vi "Z900_navX_InternalOpen.vi"(8 "error in":errorcluster, 11 "navX Device":T1={"Interface"={"Protocol"=enum."SERIAL", "Update Rate (4Hz-60Hz)"=4, "navX Open TypeDef"=variant}, "Notify Packet"=refnum, "Loop VI Refnum"=refnum} {"Interface"."Update Rate (4Hz-60Hz)" min=4 max=60 step=1}) -> (0 "error out":errorcluster, 2 "Interface TypeDefs":T3 {"I2CDevRef"."Device Address" format="%.0x"}, 3 "navX Device":T1={"Interface"={"Protocol"=enum."SERIAL", "Update Rate (4Hz-60Hz)"=4, "navX Open TypeDef"=variant}, "Notify Packet"=refnum, "Loop VI Refnum"=refnum} {"Interface"."Update Rate (4Hz-60Hz)" min=4 max=60 step=1})   [LabVIEW 2014, in "navX Library v2.lvlib"]
uses:
  navX Library v2.lvlib
  TypeDefs/Z900_navX_DeviceTypeDef.ctl
  TypeDefs/Z900_navX_ProtocolTypeDef.ctl
  TypeDefs/Z900_navX_NotifyPacketTypeDef.ctl
  TypeDefs/Z900_navX_ActionTypeDef.ctl
  TypeDefs/Z900_navX_InterfaceTypeDef.ctl
  <vilib>/Rock Robotics/WPI/SerialPort/WPI_SerialPortRef.ctl
  <vilib>/Rock Robotics/WPI/I2C/WPI_I2CDevRef.ctl
  <vilib>/Rock Robotics/SystemInterfaces/Typedef/FPGA_TypedefDigitalModule.ctl
  <vilib>/Rock Robotics/SystemInterfaces/i2clib/i2c_bus.ctl
  <vilib>/Rock Robotics/WPI/SPI/WPI_SPIDevRef.ctl
  <vilib>/Rock Robotics/SystemInterfaces/spilib/spi_bus.ctl
  TypeDefs/navX Open TypeDefs/Z900_navX_SerialOpenTypeDef.ctl
  NI WPI/WPI_SerialPort_USB.ctl
  TypeDefs/navX Open TypeDefs/Z900_navX_I2COpenTypeDef.ctl
  TypeDefs/navX Open TypeDefs/Z900_navX_SPIOpenTypeDef.ctl
  NI WPI/NI WPI Serial USB.lvlib
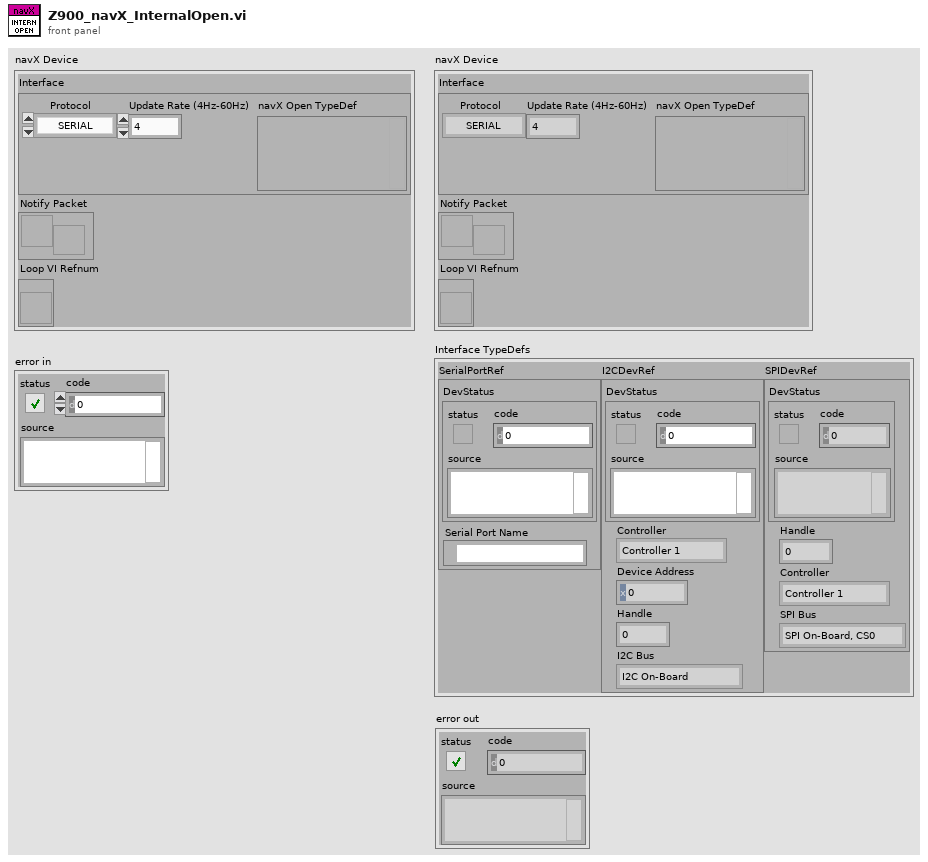
[diagram p1: front panel]
types:
  T1 = typedef "navX Library v2.lvlib/Z900_navX_DeviceTypeDef.ctl" = cluster{"Interface":cluster{"Protocol":T2, "Update Rate (4Hz-60Hz)":u8, "navX Open TypeDef":variant}, "Notify Packet":refnum<notifier>, "Loop VI Refnum":refnum<vi>}
  T2 = typedef "navX Library v2.lvlib/Z900_navX_ProtocolTypeDef.ctl" = enum16{"SERIAL", "I2C", "SPI"}
  T3 = typedef "navX Library v2.lvlib/Z900_navX_InterfaceTypeDef.ctl" = cluster{"SerialPortRef":T4, "I2CDevRef":T5, "SPIDevRef":T8}
  T4 = typedef "WPI_SerialPortRef.ctl" = cluster{"DevStatus":errorcluster, "Serial Port Name":refnum<visa-resource-name>}
  T5 = typedef "WPI_I2CDevRef.ctl" = cluster{"DevStatus":errorcluster, "Controller":T6, "Device Address":u8, "Handle":i32, "I2C Bus":T7}
  T6 = typedef "FPGA_TypedefDigitalModule.ctl" = enum16{"Controller 1"}
  T7 = typedef "i2c_bus.ctl" = enum16{"I2C On-Board", "I2C MXP", "Invalid"}
  T8 = typedef "WPI_SPIDevRef.ctl" = cluster{"DevStatus":errorcluster, "Handle":i32, "Controller":T6, "SPI Bus":T9}
  T9 = typedef "spi_bus.ctl" = enum16{"SPI On-Board, CS0", "SPI On-Board, CS1", "SPI On-Board, CS2", "SPI On-Board, CS3", "SPI MXP", "Invalid"}
  T10 = typedef "navX Library v2.lvlib/Z900_navX_SerialOpenTypeDef.ctl" = cluster{"Serial Port":T11, "Raw Data":bool}
  T11 = typedef "NI WPI Serial USB.lvlib/WPI_SerialPort_USB.ctl" = enum16{"Onboard RS-232", "MXP TTL", "USB"}
  T12 = typedef "navX Library v2.lvlib/Z900_navX_I2COpenTypeDef.ctl" = cluster{"I2C Bus":T7}
  T13 = typedef "navX Library v2.lvlib/Z900_navX_SPIOpenTypeDef.ctl" = cluster{"SPI Bus":T9}
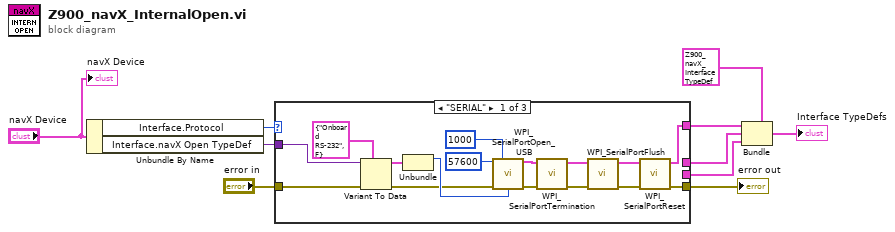
[diagram p0: block diagram]
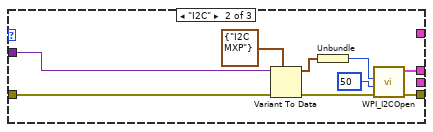
[diagram p2: hidden frame]
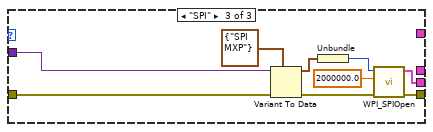
[diagram p3: hidden frame]
diagram:
  n1 = Unbundle By Name("navX Device") -> ("Interface.Protocol"=w7:T2, "Interface.navX Open TypeDef"=w6:variant)
  n2 = case shown="\"SERIAL\"" w7 {
    tunnel: w6 -> [w26 w34 w43]
    tunnel: [w14 _ _] -> w10
    tunnel: [w13 w30 w39] -> w5
    tunnel: [_ w29 _] -> w9
    tunnel: [_ _ w38] -> w8
    tunnel: "error in" -> [w12 w27 w37]
    frame "SERIAL" {
      n3 = Variant To Data(error in=w12, type=T10 {"Serial Port"=enum."Onboard RS-232", "Raw Data"=FALSE} ("navX Serial Open"), Variant=w26) -> (data=w24:T10, error out=w11:errorcluster)
      n4 = Unbundle(w24) -> ("Serial Port"=w23:T11)  [unwired: 1 out]
      n5 = call "WPI_SerialPortOpen_USB.vi"("Baud Rate"=u32 57600, "Timeout Value (ms)"=u32 1000, "error in (no error)"=w11, "Serial Port"=w23) -> ("SerialPortRef"=w16:T4, "error out"=w15:errorcluster)  [unwired: 10 in]
      n6 = call <vilib>:"WPI_SerialPortTermination.vi"("error in (no error)"=w15, "SerialPortRef"=w16) -> ("error out"=w20:errorcluster, "SerialPortRef"=w19:T4)  [unwired: 8 in]
      n7 = call <vilib>:"WPI_SerialPortFlush.vi"("error in (no error)"=w20, "SerialPortRef"=w19) -> ("error out"=w17:errorcluster, "SerialPortRef"=w18:T4)  [unwired: 8 in]
      n8 = call <vilib>:"WPI_SerialPortReset.vi"("error in (no error)"=w17, "SerialPortRef"=w18) -> ("error out"=w13:errorcluster, "SerialPortRef"=w14:T4)  [unwired: 8 in]
    }
    frame "I2C" {
      n9 = Variant To Data(error in=w27, type=T12 {"I2C Bus"=enum."I2C MXP"} ("navX I2C Open"), Variant=w34) -> (data=w35:T12, error out=w28:errorcluster)
      n10 = Unbundle(w35) -> ("I2C Bus"=w32:T7)
      n11 = call <vilib>:"WPI_I2COpen.vi"("error in"=w28, "Device Address"=u8 50, "I2C Bus"=w32) -> ("error out"=w30:errorcluster, "I2CDevRef"=w29:T5)  [unwired: 7 in]
    }
    frame "SPI" {
      n12 = Variant To Data(error in=w37, type=T13 {"SPI Bus"=enum."SPI MXP"} ("navX SPI Open"), Variant=w43) -> (data=w44:T13, error out=w36:errorcluster)
      n13 = Unbundle(w44) -> ("SPI Bus"=w41:T9)
      n14 = call <vilib>:"WPI_SPIOpen.vi"("error in"=w36, "Clock Rate (Hz)"=2000000.0, "SPI Bus"=w41) -> ("error out"=w39:errorcluster, "SPIDevRef"=w38:T8)  [unwired: 7 in]
    }
  }
  "error out" <- w5
  n15 = Bundle(cluster=T3 {"SerialPortRef"={"DevStatus"={"status"=FALSE, "code"=0, "source"=""}, "Serial Port Name"=""}, "I2CDevRef"={"DevStatus"={"status"=FALSE, "code"=0, "source"=""}, "Controller"=enum."Controller 1", "Device Address"=0, "Handle"=0, "I2C Bus"=enum."I2C On-Board"}, "SPIDevRef"={"DevStatus"={"status"=FALSE, "code"=0, "source"=""}, "Handle"=0, "Controller"=enum."Controller 1", "SPI Bus"=enum."SPI On-Board, CS0"}} ("Interface TypeDefs"), "SerialPortRef"=w10, "I2CDevRef"=w9, "SPIDevRef"=w8) -> (→"Interface TypeDefs":T3)
  "navX Device" <- "navX Device"
